vi "Create File with Incrementing Suffix [NIW].vi"(6 "disable buffering (F)":bool, 7 "format string (\" (%03d)\")":string=" (%03d)", 8 "error in (no error)":errorcluster, 11 "file path":path=path "C:/temp/test.dat") -> (0 "error out":errorcluster, 1 "File number text":string=" (001)", 2 "actual path":path=path "C:/temp/test (001).dat", 3 "refnum out":refnum<file>)   [LabVIEW 2018]
doc: "Nicolas Weiss - EPFL 2019\n\nCreates a file and appends an incrementing number suffix to the filename if the file already exists at a specified path. If the file does not exist, this VI creates the file without appending an incrementing number suffix to the filename."
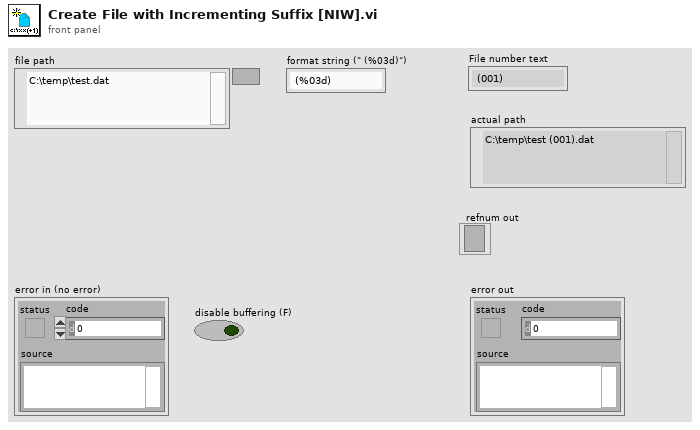
[diagram p1: front panel]
types:
  T1 = enum16{"open", "replace", "create", "open or create", "replace or create", "replace or create with confirmation"}
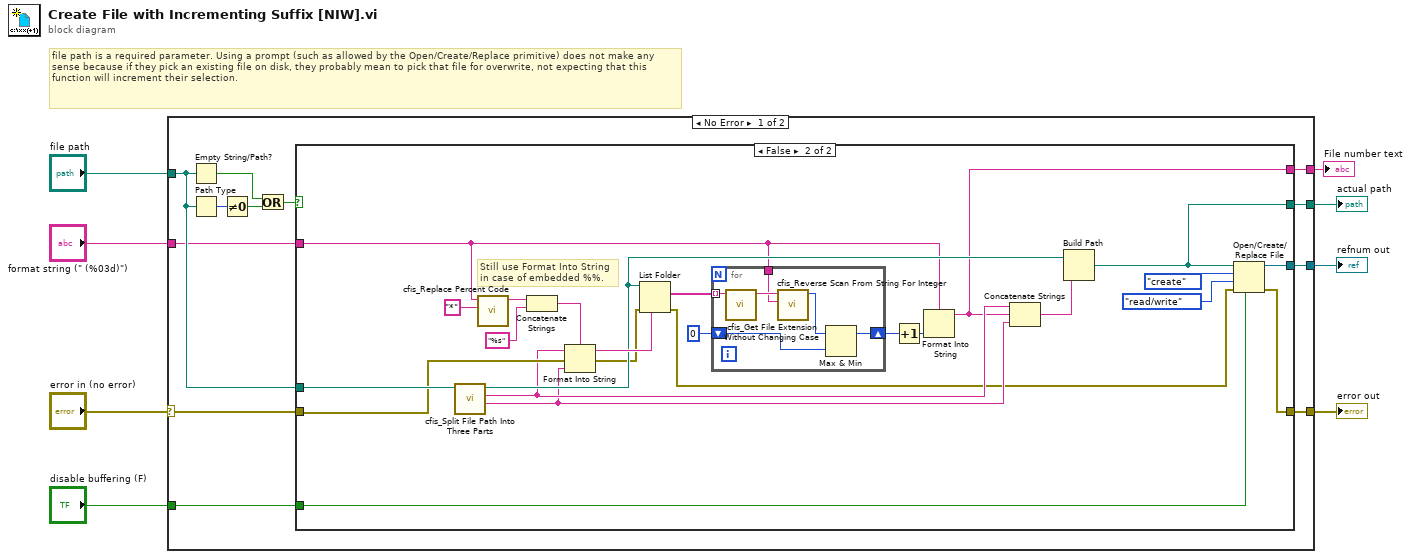
[diagram p0: block diagram]
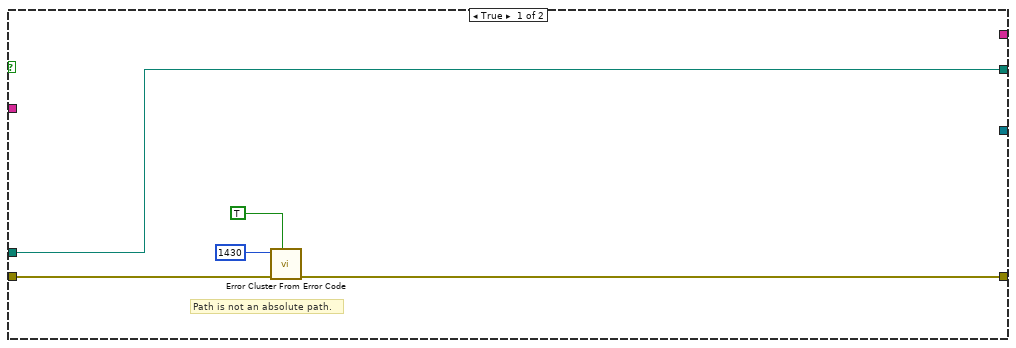
[diagram p2: hidden frame]
diagram:
  # "file path is a required parameter. Using a prompt (such as allowed by the Open/Create/Replace primitive) does not make any sense because if they pick an existing file on disk, they probably mean to pick that file for overwrite, not expecting that this function will increment their selection."
  n1 = case shown="No Error" "error in (no error)" {
    selector: "error in (no error)" -> [w17 w58]
    tunnel: "file path" -> [w12 w57]
    tunnel: "disable buffering (F)" -> [w20 _]
    tunnel: [w19 w58] -> w6
    tunnel: [w18 _] -> w2
    tunnel: [w11 w57] -> w4
    tunnel: "format string (\" (%03d)\")" -> [w10 _]
    tunnel: [w9 _] -> w1
    frame No Error {
      n2 = Empty String/Path?(string/path=w12) -> (empty?=w14:bool)
      n3 = Path Type(1:w12) -> (0:w16:i16)
      n4 = Not Equal To 0?(x=w16) -> (x != 0?=w15:bool)
      n5 = Or(x=w14, y=w15) -> (x .or. y?=w13:bool)
      n6 = case shown="False" w13 {
        tunnel: w20 -> [_ w50]
        tunnel: [w25 w49] -> w19
        tunnel: [_ w48] -> w18
        tunnel: w17 -> [w23 w33]
        tunnel: w12 -> [w21 w34]
        tunnel: [w21 w45] -> w11
        tunnel: w10 -> [_ w31]
        tunnel: [_ w26] -> w9
        frame True {
          # "Path is not an absolute path."
          n7 = call <vilib>:"Error Cluster From Error Code.vi"("show call chain? (False)"=TRUE, "error in (no error)"=w23, "error code (0)"=1430) -> ("error out"=w25:errorcluster)  [unwired: 6 in]
        }
        frame False {
          # "Still use Format Into String\nin case of embedded %%."
          n8 = call <vilib>:"cfis_Split File Path Into Three Parts.vi"("file path"=w34) -> ("File extension"=w29:string, "File name without extension"=w30:string, "Directory"=w39:path)  [unwired: 8 in]
          n9 = call <vilib>:"cfis_Replace Percent Code.vi"("replace text"="*", "format string in"=w31) -> ("format string out"=w43:string)  [unwired: 9 in]
          n10 = Concatenate Strings(w43, "%s" ("format string")) -> (w42:string)
          n11 = Format Into String(format string=w42, initial string=w30, error in=w33, w29) -> (resulting string=w40:string, error out=w38:errorcluster)
          n12 = List Folder(path=w39, pattern=w40, error in=w38) -> (filenames=w37:string[], error out=w28:errorcluster)  [unwired: 1 in, 2 out]
          n13 = for {
            tunnel: w37 -> [w56] mode=indexing
            shift-right: [w52] -> w35
            shift-left: 0 -> [w53]
            tunnel: w31 -> [w51]
            n14 = call <vilib>:"cfis_Get File Extension Without Changing Case.vi"("file name"=w56) -> ("file name without extension"=w55:string)  [unwired: 9 in, 1 out]
            n15 = call <vilib>:"cfis_Reverse Scan From String For Integer.vi"("format string"=w51, "input string"=w55) -> ("Extracted integer"=w54:i32)  [unwired: 9 in]
            n16 = Max & Min(x=w54, y=w53) -> (max(x,y)=w52:i32)  [unwired: 1 out]
          }
          n17 = Increment(x=w35) -> (x+1=w32:i32)
          n18 = Format Into String(format string=w31, w32) -> (resulting string=w26:string)  [unwired: 2 in, 1 out]
          n19 = Concatenate Strings(w30, w26, w29) -> (w27:string)
          n20 = Build Path(base path=w39, name or relative path=w27) -> (appended path=w45:path)
          n21 = Open/Create/Replace File(file path (use dialog)=w45, error in=w28, operation (0:open)=T1."create", access (0:read/write)=enum16{"read/write", "read-only", "write-only"}."read/write", disable buffering (F)=w50) -> (refnum out=w48:refnum<file>, error out=w49:errorcluster)  [unwired: 1 in, 1 out]
        }
      }
    }
    frame Error {
    }
  }
  "error out" <- w6
  "refnum out" <- w2
  "actual path" <- w4
  "File number text" <- w1
